vi "process_pockels.vi"() -> ()   [LabVIEW 2011, in "Fiberscope_library.lvlib"]
uses:
  Fiberscope_library.lvlib
  typedefs/control_process_state_cluster.ctl
  typedefs/control_process_state_enum.ctl
  typedefs/feedback_to_watchdog.ctl
  typedefs/feedback_from_process_enum.ctl
  typedefs/pockels_calibration_cluster.ctl
  typedefs/all_scan_parameters_cluster.ctl
  typedefs/fiber_parameters_cluster.ctl
  fpga/typedefs/ramp_type_enum.ctl
  typedefs/spiral_parameters_cluster.ctl
  typedefs/run_parameters_cluster.ctl
  typedefs/run_mode_enum.ctl
  typedefs/acquisition_parameters_cluster.ctl
  typedefs/image_size_I32.ctl
  typedefs/smooth_coeffs_cluster.ctl
  typedefs/storage_parameters_cluster.ctl
  typedefs/mapping_corrections_cluster.ctl
  typedefs/pockels_corrections_cluster.ctl
  <vilib>/DAQmx/write.llb/DAQmx Write (Analog 1D DBL 1Chan NSamp).vi
  <vilib>/DAQmx/create/channels.llb/DAQmx Create Channel (AO-Voltage-Basic).vi
  <vilib>/DAQmx/configure/timing.llb/DAQmx Timing (Sample Clock).vi
  <vilib>/DAQmx/configure/trigger.llb/DAQmx Start Trigger (Digital Edge).vi
  <vilib>/DAQmx/miscellaneous.llb/DAQmx Fill In Error Info.vi
panel:
  out "Power estimate":dbl caption="[mW]"
  out "Local exit":bool
  in  "PockelsVolt":dbl(slide) min=0.0 max=1.0 step=0.005 scale=0.0..1.0
  out "error out":errorcluster
  in  "error in":errorcluster
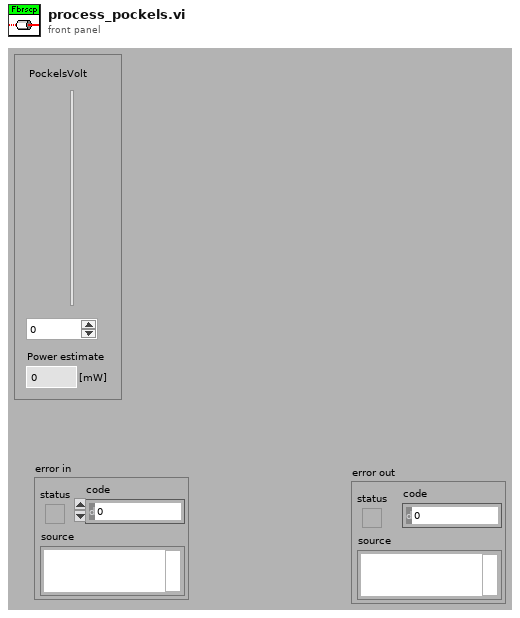
[diagram p1: front panel]
types:
  T1 = typedef "Fiberscope_library.lvlib/pockels_calibration_cluster.ctl" = cluster{"y0":dbl, "A":dbl, "w":dbl, "phi":dbl}
  T2 = typedef "Fiberscope_library.lvlib/feedback_to_watchdog.ctl" = cluster{"Feedback_from_process_enum":T3, "Process_name":string}
  T3 = typedef "Fiberscope_library.lvlib/feedback_from_process_enum.ctl" = enum16{"Has_initialised", "Changed_parameters", "Has_started", "Has_stopped", "Has_quitted", "Is_running", "Has_finished", "Custom"}
  T4 = typedef "Fiberscope_library.lvlib/control_process_state_cluster.ctl" = cluster{"Control_process_state_enum":T5, "variant":variant}
  T5 = typedef "Fiberscope_library.lvlib/control_process_state_enum.ctl" = enum16{"Init", "Quit", "Start", "Stop", "Change_parameters", "Running", "Finish", "Custom"}
  T6 = typedef "Fiberscope_library.lvlib/all_scan_parameters_cluster.ctl" = cluster{"Fiber parameters":T7, "Spiral parameters":T9, "Run parameters":T10, "Acquisition parameters":T12, "Fiber parameters pixel_mapper":T7, "Smooth_coeffs_cluster":T14, "Storage parameters":T15, "Mapping corrections":T16, "Pockels corrections":T17}
  T7 = typedef "Fiberscope_library.lvlib/fiber_parameters_cluster.ctl" = cluster{"Frequency":dbl, "Amplitude X":dbl, "Amplitude Y":dbl, "Initial Amplitude X":dbl, "Initial Amplitude Y":dbl, "Phase":dbl, "Ramp type":T8}
  T8 = typedef "ramp_type_enum.ctl" = enum8{"Linear", "Sine"}
  T9 = typedef "Fiberscope_library.lvlib/spiral_parameters_cluster.ctl" = cluster{"Imaging periods":dbl, "Settling periods":dbl, "Resting periods":dbl}
  T10 = typedef "Fiberscope_library.lvlib/run_parameters_cluster.ctl" = cluster{"Run mode":T11, "Averages per frame":u8, "No. of frames":u32}
  T11 = typedef "Fiberscope_library.lvlib/run_mode_enum.ctl" = enum16{"Continuous", "Single frame", "No. of frames"}
  T12 = typedef "Fiberscope_library.lvlib/acquisition_parameters_cluster.ctl" = cluster{"Cycles per pixel":u32, "Image size":T13, "Bidirectional acquisition":bool}
  T13 = typedef "Fiberscope_library.lvlib/image_size_I32.ctl" = i32
  T14 = typedef "Fiberscope_library.lvlib/smooth_coeffs_cluster.ctl" = cluster{"Coeff 1":dbl, "Coeff 2":dbl}
  T15 = typedef "Fiberscope_library.lvlib/storage_parameters_cluster.ctl" = cluster{"Autosave":bool, "Path":path}
  T16 = typedef "Fiberscope_library.lvlib/mapping_corrections_cluster.ctl" = cluster{"Phase increase":dbl, "Amplitude correction":dbl}
  T17 = typedef "Fiberscope_library.lvlib/pockels_corrections_cluster.ctl" = cluster{"Delay pixels":i32}
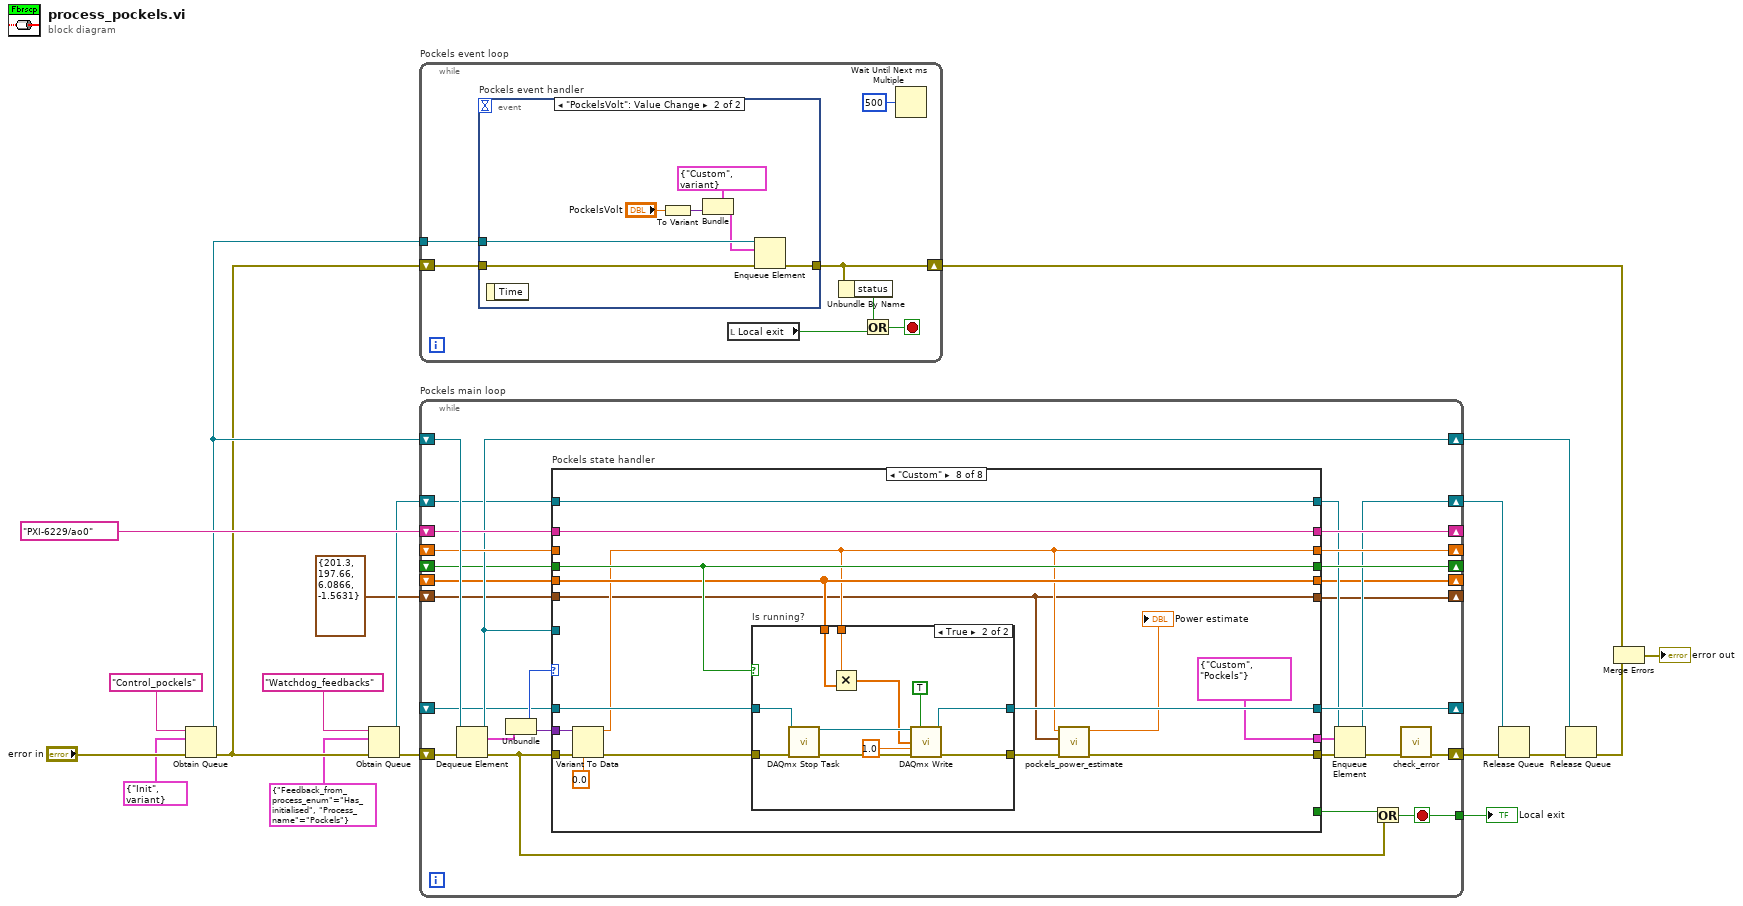
[diagram p0: block diagram]
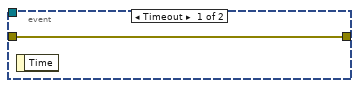
[diagram p2: hidden frame]
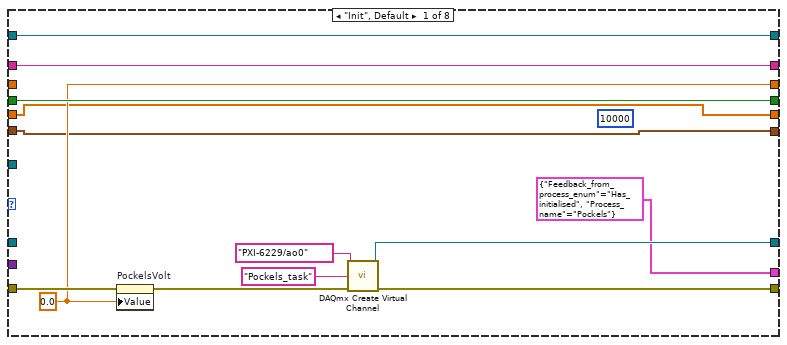
[diagram p3: hidden frame]
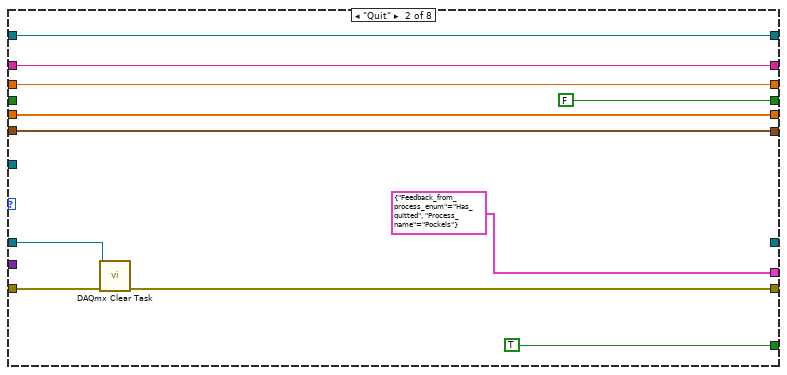
[diagram p4: hidden frame]
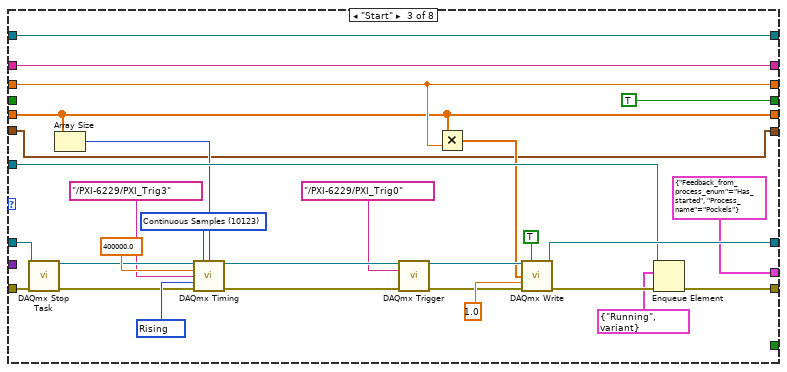
[diagram p5: hidden frame]
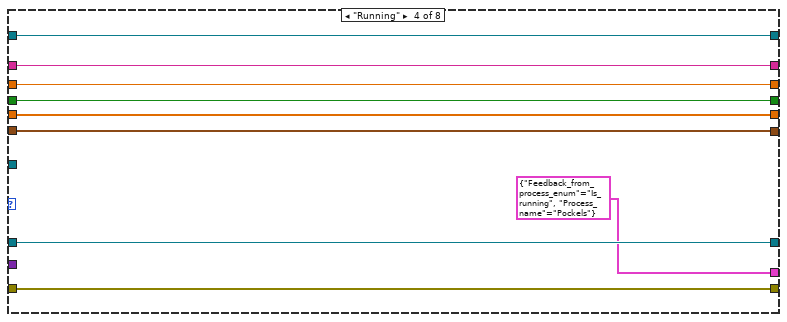
[diagram p6: hidden frame]
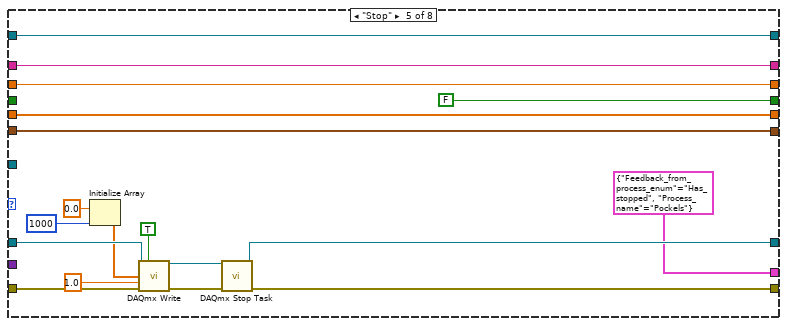
[diagram p7: hidden frame]
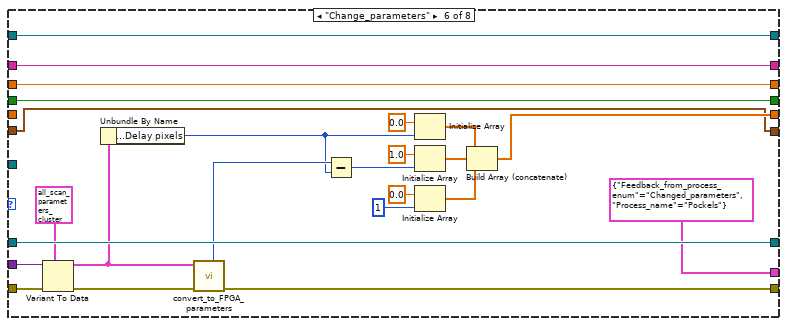
[diagram p8: hidden frame]
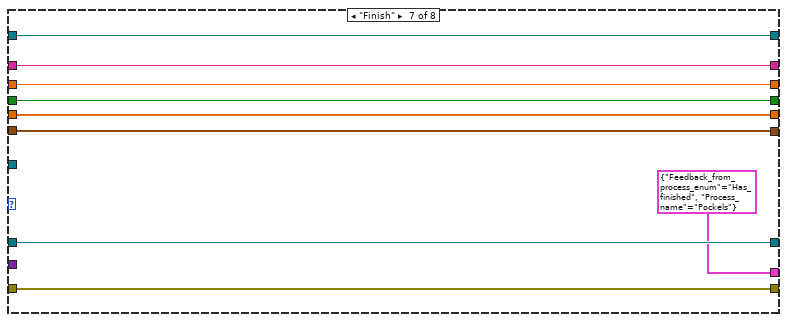
[diagram p9: hidden frame]
diagram:
  n1 = Obtain Queue(name (unnamed)="Control_pockels", element data type=T4 {"Control_process_state_enum"=enum."Init", "variant"=variant} ("Control_process_state_cluster"), error in (no error)="error in") -> (queue out=w8:refnum<queue>, error out=w7:errorcluster)  [unwired: 2 in, 1 out]
  n2 = Obtain Queue(name (unnamed)="Watchdog_feedbacks", element data type=T2 {"Feedback_from_process_enum"=enum."Has_initialised", "Process_name"="Pockels"}, error in (no error)=w7) -> (queue out=w12:refnum<queue>, error out=w14:errorcluster)  [unwired: 2 in, 1 out]
  n3 = while "Pockels event loop" {
    shift-right: [w24] -> w5
    shift-left: w7 -> [w25]
    tunnel: w8 -> [w26]
    stop <- w22 stop-if-true
    n4 = event "Pockels event handler" shown="[1] \"PockelsVolt\": Value Change" {
      selector: _ -> [_ _]
      dyn-events: _ -> [_ _]
      timeout: _ -> [_ _]
      tunnel: w26 -> [_ w33]
      tunnel: w25 -> [w27 w34]
      tunnel: [w27 w32] -> w24
      event Timeout {
        n5 = event-data() -> ()  [unwired: 1 in, 1 out]
      }
      event "PockelsVolt": Value Change {
        n6 = event-data() -> ()  [unwired: 1 in, 1 out]
        n7 = To Variant(anything="PockelsVolt") -> (Variant=w29:variant)
        n8 = Bundle(cluster=T4 {"Control_process_state_enum"=enum."Custom", "variant"=variant} ("Control_process_state_cluster"), "variant"=w29) -> (w31:T4)  [unwired: 1 in]
        n9 = Enqueue Element(queue=w33, element=w31, error in (no error)=w34) -> (error out=w32:errorcluster)  [unwired: 1 in, 2 out]
      }
    }
    n10 = local read "Local exit"() -> (w21:bool)
    n11 = Unbundle By Name(w24) -> ("status"=w23:bool)
    n12 = Or(x=w23, y=w21) -> (x .or. y?=w22:bool)
    n13 = Wait Until Next ms Multiple(millisecond multiple=u32 500) -> ()  [unwired: 1 out]
  }
  n14 = while "Pockels main loop" {
    shift-right: [w57] -> w11
    shift-left: w14 -> [w62]
    shift-right: [w52] -> w16
    shift-left: w8 -> [w61]
    shift-right: [w55] -> _
    shift-left: tag "PXI-6229/ao0" ("physical channels") -> [w56]
    shift-right: [w54] -> _
    shift-left: _ -> [w53]
    shift-right: [w51] -> _
    shift-left: _ -> [w50]
    shift-right: [w39] -> w9
    shift-left: w12 -> [w49]
    shift-right: [w48] -> _
    shift-left: _ -> [w47]
    tunnel: [w46] -> w6
    shift-right: [w38] -> _
    shift-left: _ -> [w37]
    shift-right: [w36] -> _
    shift-left: T1 {"y0"=201.3, "A"=197.66, "w"=6.0866, "phi"=-1.5631} ("Pockels calibration") -> [w35]
    stop <- w46 stop-if-true
    n15 = Dequeue Element(queue=w61, error in (no error)=w62) -> (queue out=w52:refnum<queue>, element=w60:T4, error out=w41:errorcluster)  [unwired: 1 in, 1 out]
    n16 = Unbundle(w60) -> ("Control_process_state_enum"=w59:T5, "variant"=w58:variant)
    n17 = case "Pockels state handler" shown="\"Custom\"" w59 {
      tunnel: w41 -> [w70 w83 w110 w124 w134 w160 w175 w190]
      tunnel: [w67 w80 w101 w124 w138 w151 w175 w179] -> w45
      tunnel: w58 -> [_ _ _ _ _ w159 _ w189]
      tunnel: [_ TRUE _ _ _ _ _ _] -> w42
      tunnel: w56 -> [w75 w85 w113 w123 w142 w166 w174 w191]
      tunnel: [w75 w85 w113 w123 w142 w166 w174 w191] -> w55
      tunnel: [w68 w84 w91 w122 w141 w165 w173 w177] -> w54
      tunnel: w53 -> [_ w84 w91 w122 w141 w165 w173 _]
      tunnel: w52 -> [_ _ w100 _ _ _ _ _]
      tunnel: [w71 _ w105 w121 w140 w164 w172 w187] -> w51
      tunnel: w50 -> [_ w82 w108 w121 w131 w164 w172 w185]
      tunnel: [w66 w79 w103 w120 w137 w163 w171 w183] -> w43
      tunnel: w49 -> [w66 w79 w103 w120 w137 w163 w171 w183]
      tunnel: [w72 FALSE TRUE w119 FALSE w162 w170 w184] -> w48
      tunnel: w47 -> [w72 _ _ w119 _ w162 w170 w184]
      tunnel: [T2 {"Feedback_from_process_enum"=enum."Has_initialised", "Process_name"="Pockels"} T2 {"Feedback_from_process_enum"=enum."Has_quitted", "Process_name"="Pockels"} T2 {"Feedback_from_process_enum"=enum."Has_started", "Process_name"="Pockels"} T2 {"Feedback_from_process_enum"=enum."Is_running", "Process_name"="Pockels"} T2 {"Feedback_from_process_enum"=enum."Has_stopped", "Process_name"="Pockels"} T2 {"Feedback_from_process_enum"=enum."Changed_parameters", "Process_name"="Pockels"} T2 {"Feedback_from_process_enum"=enum."Has_finished", "Process_name"="Pockels"} T2 {"Feedback_from_process_enum"=enum."Custom", "Process_name"="Pockels"}] -> w40
      tunnel: [w64 w77 w89 w117 w135 w153 w168 w181] -> w38
      tunnel: w37 -> [w64 w77 w89 w117 w135 _ w168 w181]
      tunnel: w35 -> [w63 w76 w87 w116 w125 w143 w167 w176]
      tunnel: [w63 w76 w87 w116 w125 w143 w167 w176] -> w36
      frame "Init", Default {
        (unwired) 10000 ("dimension size")
        w68 = 0.0
        n18 = property on="PockelsVolt" class="Slide (strict)"(error in=w70, "Value"=w68) -> (error out=w69:errorcluster)  [unwired: 1 in, 1 out]
        n19 = call-poly <vilib>:"DAQmx Create Virtual Channel.vi"("physical channels"=tag "PXI-6229/ao0", "name to assign"="Pockels_task", "error in"=w69) -> ("task out"=w71:refnum<k21>, "error out"=w67:errorcluster)  [unwired: 11 in]
      }
      frame "Quit" {
        n20 = call <vilib>:"DAQmx Clear Task.vi"("task in"=w82, "error in"=w83) -> ("error out"=w80:errorcluster)  [unwired: 13 in]
      }
      frame "Start" {
        w112 = 10123 items=["Finite Samples"=10178, "Continuous Samples"=10123, "Hardware Timed Single Point"=12522] ("sample mode")
        w115 = 10280 items=["Rising"=10280, "Falling"=10171] ("active edge")
        n21 = call <vilib>:"DAQmx Stop Task.vi"("task/channels in"=w108, "error in"=w110) -> ("task out"=w107:refnum<k21>, "error out"=w109:errorcluster)  [unwired: 12 in]
        n22 = Array Size(array=w89) -> (size(s)=w88:i32)
        n23 = call-poly <vilib>:"DAQmx Timing.vi"("task/channels in"=w107, "sample mode"=w112, "samples per channel"=w88, "rate"=400000.0, "source"=tag "/PXI-6229/PXI_Trig3", "active edge"=w115, "error in"=w109) -> ("task out"=w96:refnum<k21>, "error out"=w95:errorcluster)  [unwired: 7 in]
        n24 = call-poly <vilib>:"DAQmx Trigger.vi"("task/channels in"=w96, "source"=tag "/PXI-6229/PXI_Trig0", "error in"=w95) -> ("task out"=w92:refnum<k21>, "error out"=w93:errorcluster)  [unwired: 11 in]
        n25 = Multiply(x=w89, y=w91) -> (x*y=w90:dbl[])
        n26 = call-poly <vilib>:"DAQmx Write.vi"("task/channels in"=w92, "auto start"=TRUE, "data"=w90, "timeout"=1.0, "error in"=w93) -> ("task out"=w105:refnum<k21>, "error out"=w102:errorcluster)  [unwired: 8 in, 1 out]
        n27 = Enqueue Element(queue=w100, element=T4 {"Control_process_state_enum"=enum."Running", "variant"=variant}, error in (no error)=w102) -> (error out=w101:errorcluster)  [unwired: 1 in, 2 out]
      }
      frame "Running" {
      }
      frame "Stop" {
        n28 = Initialize Array(0.0 ("element"), 1000 ("dimension size")) -> (w129:dbl[])
        n29 = call-poly <vilib>:"DAQmx Write.vi"("task/channels in"=w131, "auto start"=TRUE, "data"=w129, "timeout"=1.0, "error in"=w134) -> ("task out"=w132:refnum<k21>, "error out"=w133:errorcluster)  [unwired: 8 in, 1 out]
        n30 = call <vilib>:"DAQmx Stop Task.vi"("task/channels in"=w132, "error in"=w133) -> ("task out"=w140:refnum<k21>, "error out"=w138:errorcluster)  [unwired: 12 in]
      }
      frame "Change_parameters" {
        n31 = Variant To Data(error in=w160, type=T6 {"Fiber parameters"={"Frequency"=100.0, "Amplitude X"=0.0, "Amplitude Y"=0.0, "Initial Amplitude X"=0.0, "Initial Amplitude Y"=0.0, "Phase"=0.0, "Ramp type"=enum."Linear"}, "Spiral parameters"={"Imaging periods"=1.0, "Settling periods"=1.0, "Resting periods"=1.0}, "Run parameters"={"Run mode"=enum."Continuous", "Averages per frame"=0, "No. of frames"=0}, "Acquisition parameters"={"Cycles per pixel"=0, "Image size"=1, "Bidirectional acquisition"=FALSE}, "Fiber parameters pixel_mapper"={"Frequency"=0.0, "Amplitude X"=0.0, "Amplitude Y"=0.0, "Initial Amplitude X"=0.0, "Initial Amplitude Y"=0.0, "Phase"=0.0, "Ramp type"=enum."Linear"}, "Smooth_coeffs_cluster"={"Coeff 1"=0.0, "Coeff 2"=0.0}, "Storage parameters"={"Autosave"=FALSE, "Path"=path ""}, "Mapping corrections"={"Phase increase"=0.0, "Amplitude correction"=0.0}, "Pockels corrections"={"Delay pixels"=0}} ("All scan parameters"), Variant=w159) -> (data=w149:T6, error out=w152:errorcluster)
        n32 = Unbundle By Name(w149) -> ("Pockels corrections.Delay pixels"=w144:i32)
        n33 = call "convert_to_FPGA_parameters.vi"("error in"=w152, "All scan parameters"=w149) -> ("error out"=w151:errorcluster, "Pixels per spiral"=w145:i32)  [unwired: 4 in, 4 out]
        n34 = Subtract(x=w145, y=w144) -> (x-y=w146:i32)
        n35 = Initialize Array(0.0 ("element"), w144) -> (w148:dbl[])
        n36 = Initialize Array(1.0 ("element"), w146) -> (w155:dbl[])
        n37 = Initialize Array(0.0 ("element"), 1 ("dimension size")) -> (w154:dbl[])
        n38 = Build Array (concatenate)(w148, w155, w154) -> (w153:dbl[])
      }
      frame "Finish" {
      }
      frame "Custom" {
        n39 = Variant To Data(error in=w190, type=0.0, Variant=w189) -> (data=w177:dbl, error out=w186:errorcluster)
        n40 = case "Is running?" shown="True" w184 {
          tunnel: [w192 w204] -> w180
          tunnel: [w193 w203] -> w187
          tunnel: w177 -> [_ w196]
          tunnel: w186 -> [w192 w200]
          tunnel: w185 -> [w193 w197]
          tunnel: w181 -> [_ w195]
          frame False {
          }
          frame True {
            n41 = call <vilib>:"DAQmx Stop Task.vi"("task/channels in"=w197, "error in"=w200) -> ("task out"=w198:refnum<k21>, "error out"=w199:errorcluster)  [unwired: 12 in]
            n42 = Multiply(x=w196, y=w195) -> (x*y=w194:dbl[])
            n43 = call-poly <vilib>:"DAQmx Write.vi"("task/channels in"=w198, "auto start"=TRUE, "data"=w194, "timeout"=1.0, "error in"=w199) -> ("task out"=w203:refnum<k21>, "error out"=w204:errorcluster)  [unwired: 8 in, 1 out]
          }
        }
        n44 = call "pockels_power_estimate.vi"("error in"=w180, "Pockels calibration"=w176, "Pockels volt"=w177) -> ("error out"=w179:errorcluster, "Power estimate"=→"Power estimate":dbl)  [unwired: 7 in]
      }
    }
    n45 = Enqueue Element(queue=w43, element=w40, error in (no error)=w45) -> (queue out=w39:refnum<queue>, error out=w44:errorcluster)  [unwired: 1 in, 1 out]
    n46 = Or(x=w42, y=w41) -> (x .or. y?=w46:bool)
    n47 = call "check_error.vi"("error in"=w44) -> ("error out"=w57:errorcluster)  [unwired: 10 in]
  }
  "Local exit" <- w6
  n48 = Release Queue(queue=w9, error in (no error)=w11) -> (error out=w10:errorcluster)  [unwired: 1 in, 2 out]
  n49 = Release Queue(queue=w16, error in (no error)=w10) -> (error out=w4:errorcluster)  [unwired: 1 in, 2 out]
  n50 = Merge Errors(w5, w4) -> (→"error out":errorcluster)
